vi "Load AcqMode doc.vi"(11 "Mode":T1) -> (3 "new picture":picture)   [LabVIEW 2011]
uses:
  TDE_mode.ctl
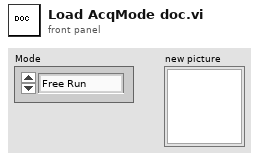
[diagram p1: front panel]
types:
  T1 = typedef "TDE_mode.ctl" = enum16{"Free Run", "ExSync Prog", "ExSync Lev", "ExSync Edge"}
  T2 = typedef "imagedata.ctl" = cluster{"image type":i32, "image depth":i32, "image":u8[], "mask":u8[], "colors":u32[], "Rectangle":cluster{"left":i16, "top":i16, "right":i16, "bottom":i16}}
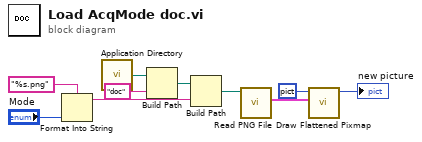
[diagram p0: block diagram]
diagram:
  n1 = Format Into String(format string="%s.png", "Mode") -> (resulting string=w5:string)  [unwired: 2 in, 1 out]
  n2 = call <vilib>:"Application Directory.vi"() -> ("Application Directory"=w3:path)
  n3 = Build Path(base path=w3, name or relative path="doc" ("format string")) -> (appended path=w2:path)
  n4 = Build Path(base path=w2, name or relative path=w5) -> (appended path=w4:path)
  n5 = call <vilib>:"Read PNG File.vi"("path to PNG file"=w4) -> ("image data"=w8:T2)  [unwired: 8 in, 2 out]
  n6 = call <vilib>:"Draw Flattened Pixmap.vi"("image data"=w8, "picture"=picture data[5B]) -> ("new picture"=→"new picture":picture)  [unwired: 7 in]
